vi "HXG2_PIDs_Array_Industrial.vi"(0 "Calculated Values":T3, 1 "PID Cluster":T7, 2 "Evap Target Delta (-°F) 2":cluster{"m":dbl, "b":dbl}={"m"=0.2667, "b"=7.333}, 3 "AIR-LIQ Cluster":T4 {"Liq Cluster"."Liq TEMP %" min=0.0 max=100.0 step=1.0 format="%#.1f"; "Liq Cluster"."Liq FLOW %" min=0.0 max=100.0 step=1.0 format="%#.1f"; "Liq Cluster"."TLiq °F" min=40.0 max=180.0 step=1.0 format="%#.1f"; "Liq Cluster"."Mdot lbm/hr" min=0.0 max=1000.0 step=1.0 format="%#.1f"; "Air Cluster"."Air TEMP %" min=0.0 max=100.0 step=1.0 format="%#.1f"; "Air Cluster"."Air FLOW %" min=0.0 max=100.0 step=1.0 format="%#.1f"; "Air Cluster"."Tair  °F" min=-5.0 max=100.0 step=1.0 format="%#.1f"; "Air Cluster"."CFMs" min=0.0 max=200.0 step=1.0 format="%#.1f"}, 4 "Tank Target Delta (+°F)":dbl, 5 "error in (no error)":errorcluster, 6 "Analog In":T2, 7 "PID Ctrls":T1) -> (14 "PID Ctrls Out":T1, 19 "error out":errorcluster)   [LabVIEW 2012]
uses:
  Controls/HXG2_PIDctrlsOUT.ctl
  Controls/HXG2_PIDCluster.ctl
  Controls/HXG2_PIDon-off.ctl
  PID/HXG2_Horizontal PID Control.ctl
  PID/HXG2_Horizontal Reset Control.ctl
  Controls/HXG2_AirGly-Cluster.ctl
  Controls/UI/HXG2_UI_ControlSetAir.ctl
  Controls/UI/HXG2_UI_ControlSetGly.ctl
  Controls/HXG2_Calculated.ctl
  Controls/HXG2_AnalogIn.ctl
  Modules/EnableAirGly/HXG2enable.ctl
  Controls/UI/HXG2_NumDisplayLarge.ctl
  <vilib>/addons/control/pid/pid.llb/PID Advanced (DBL Array).vi
  <vilib>/addons/control/pid/pid.llb/PID Derivative Action Buffered (DBL Array).vi
  <vilib>/addons/control/pid/pid.llb/PID Get Advanced Error (DBL Array).vi
  <vilib>/addons/control/pid/pid.llb/PID Integral Action Buffered (DBL Array).vi
  <vilib>/addons/control/pid/pid.llb/PID Resize 1D Array.vi
  <vilib>/addons/control/pid/pid.llb/PID Get Advanced Error (DBL).vi
  <vilib>/addons/control/pid/pid.llb/PID Control Input Filter (DBL).vi
  <vilib>/addons/control/pid/pid.llb/PID Gain Schedule (DBL).vi
  <vilib>/addons/control/pid/pid.llb/PID Parameter Manager (DBL Array).vi
  <vilib>/addons/control/pid/NI_PID_pid.lvlib
panel:
  out "index out Air":i32
  out "index out Liq":i32
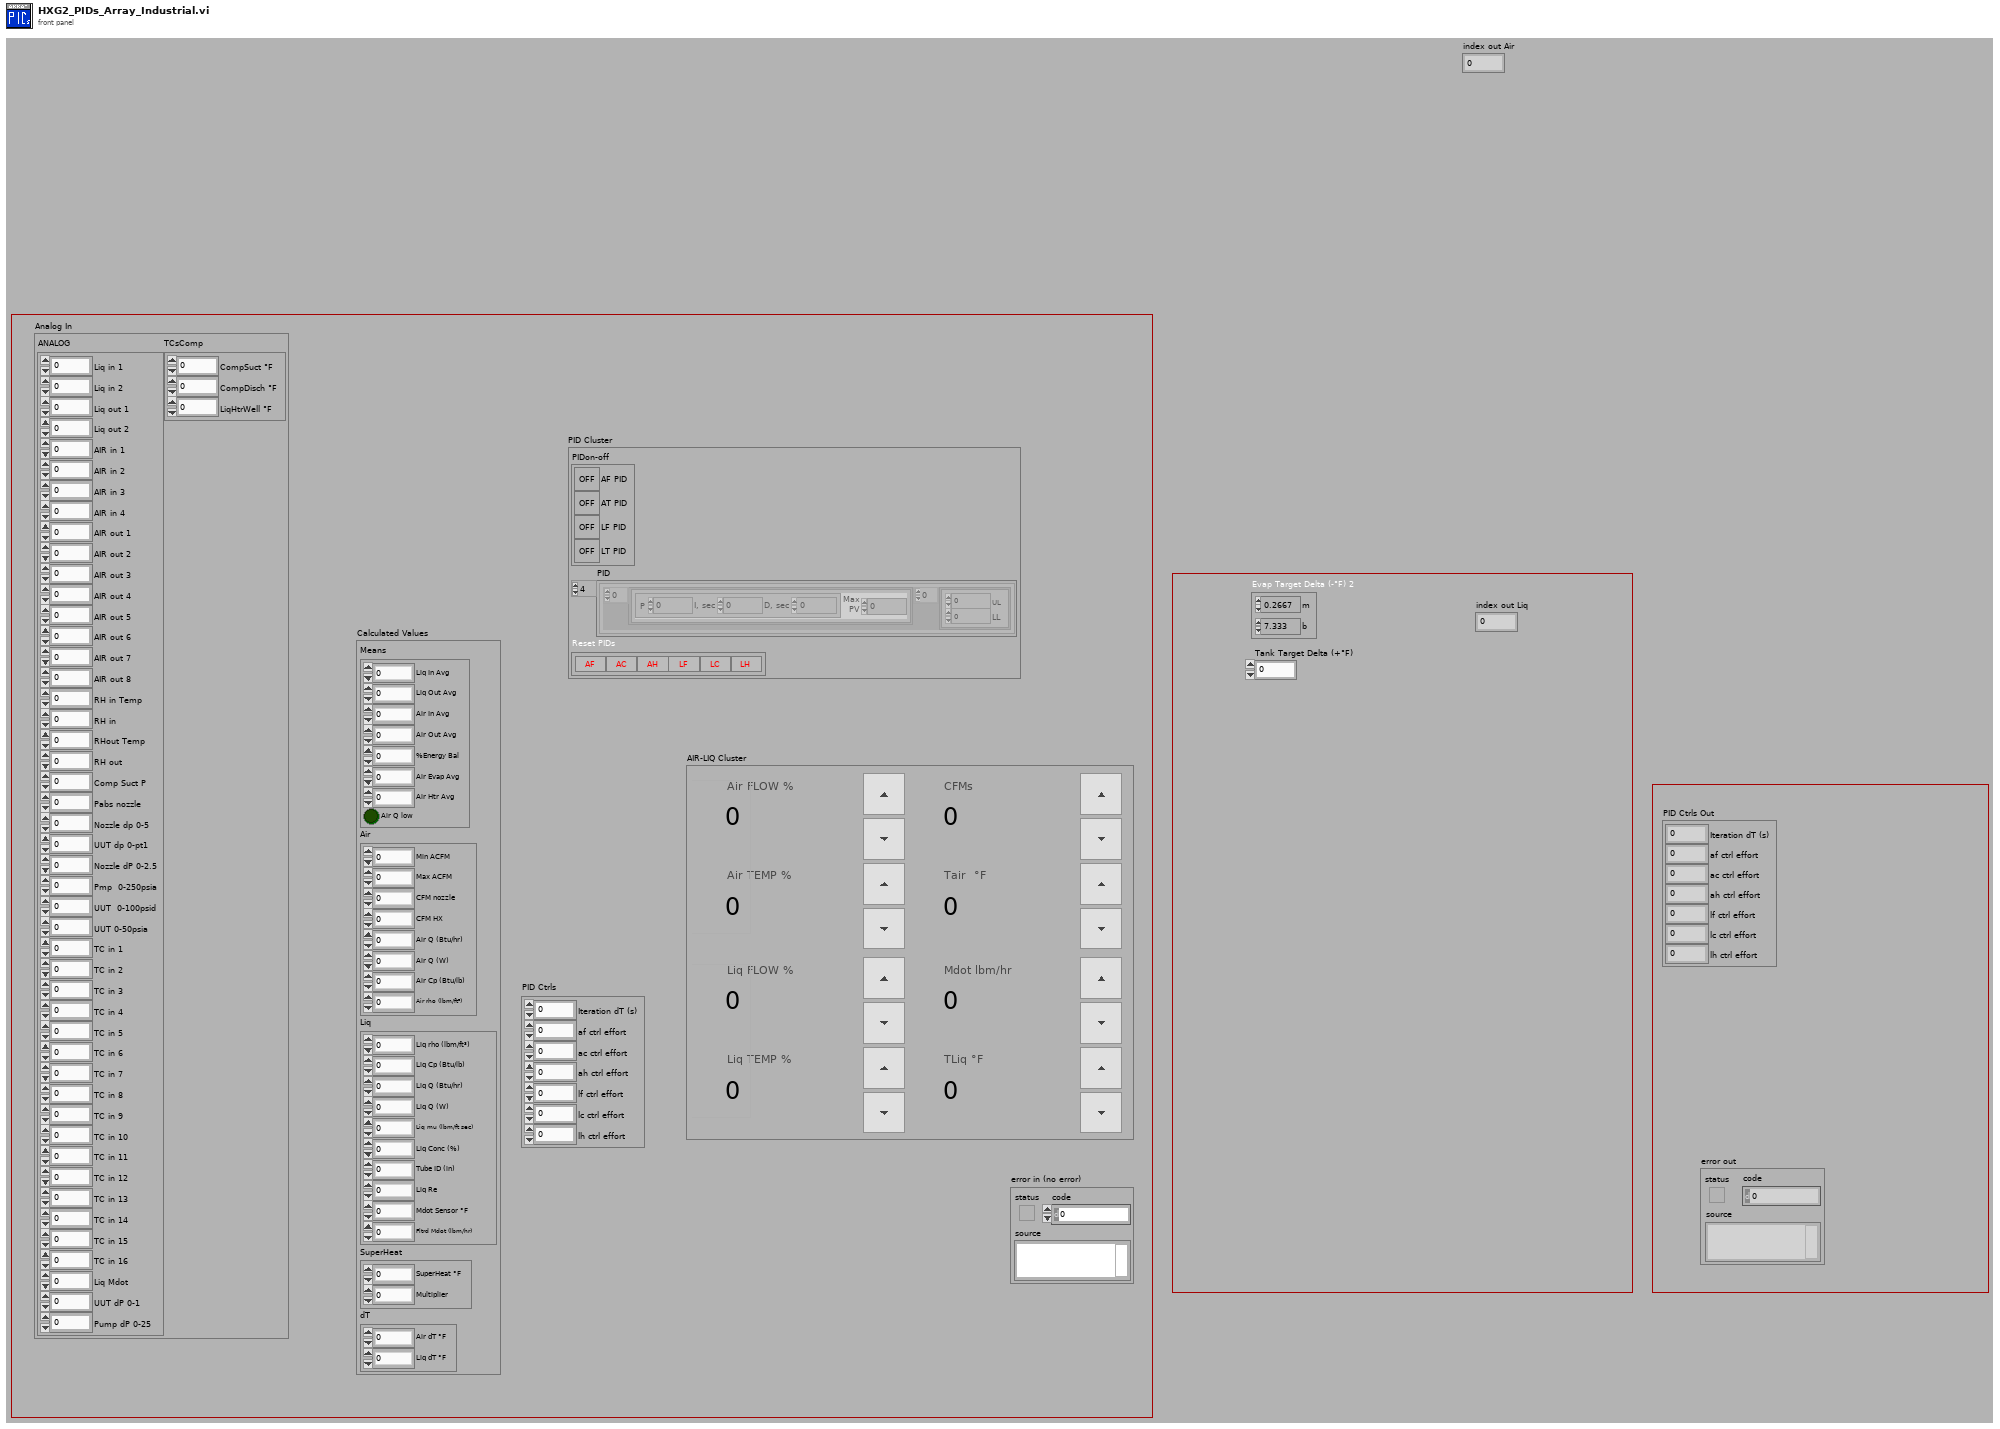
[diagram p1: front panel]
types:
  T1 = typedef "HXG2_PIDctrlsOUT.ctl" = cluster{"Iteration dT (s)":dbl, "af ctrl effort":dbl, "ac ctrl effort":dbl, "ah ctrl effort":dbl, "lf ctrl effort":dbl, "lc ctrl effort":dbl, "lh ctrl effort":dbl}
  T2 = typedef "HXG2_AnalogIn.ctl" = cluster{"ANALOG":cluster{"Liq in 1":dbl, "Liq in 2":dbl, "Liq out 1":dbl, "Liq out 2":dbl, "AIR in 1":dbl, "AIR in 2":dbl, "AIR in 3":dbl, "AIR in 4":dbl, "AIR out 1":dbl, "AIR out 2":dbl, "AIR out 3":dbl, "AIR out 4":dbl, "AIR out 5":dbl, "AIR out 6":dbl, "AIR out 7":dbl, "AIR out 8":dbl, "RH in Temp":dbl, "RH in":dbl, "RHout Temp":dbl, "RH out":dbl, "Comp Suct P":dbl, "Pabs nozzle":dbl, "Nozzle dp 0-5":dbl, "UUT dp 0-pt1":dbl, "Nozzle dP 0-2.5":dbl, "Pmp  0-250psia":dbl, "UUT  0-100psid":dbl, "UUT 0-50psia":dbl, "TC in 1":dbl, "TC in 2":dbl, "TC in 3":dbl, "TC in 4":dbl, "TC in 5":dbl, "TC in 6":dbl, "TC in 7":dbl, "TC in 8":dbl, "TC in 9":dbl, "TC in 10":dbl, "TC in 11":dbl, "TC in 12":dbl, "TC in 13":dbl, "TC in 14":dbl, "TC in 15":dbl, "TC in 16":dbl, "Liq Mdot":dbl, "UUT dP 0-1":dbl, "Pump dP 0-25":dbl}, "TCsComp":cluster{"CompSuct °F  ":dbl, "CompDisch °F":dbl, "LiqHtrWell °F":dbl}}
  T3 = typedef "HXG2_Calculated.ctl" = cluster{"Means":cluster{"Liq In Avg":dbl, "Liq Out Avg":dbl, "Air In Avg":dbl, "Air Out Avg":dbl, "%Energy Bal":dbl, "Air Evap Avg":dbl, "Air Htr Avg":dbl, "Air Q low":bool}, "Air":cluster{"Min ACFM":dbl, "Max ACFM":dbl, "CFM nozzle":dbl, "CFM HX":dbl, "Air Q (Btu/hr)":dbl, "Air Q (W)":dbl, "Air Cp (Btu/lb)":dbl, "Air rho (lbm/ft³)":dbl}, "Liq":cluster{"Liq rho (lbm/ft³)":dbl, "Liq Cp (Btu/lb)":dbl, "Liq Q (Btu/hr)":dbl, "Liq Q (W)":dbl, "Liq mu (lbm/ft sec)":dbl, "Liq Conc (%)":dbl, "Tube ID (in)":dbl, "Liq Re":dbl, "Mdot Sensor °F":dbl, "Fltrd Mdot (lbm/hr)":dbl}, "SuperHeat":cluster{"SuperHeat °F":dbl, "Multiplier":dbl}, "dT":cluster{"Air dT °F":dbl, "Liq dT °F":dbl}}
  T4 = typedef "HXG2_AirGly-Cluster.ctl" = cluster{"Air Cluster":T5, "Liq Cluster":T6}
  T5 = typedef "HXG2_UI_ControlSetAir.ctl" = cluster{"Air FLOW %":dbl, "Air TEMP % ":dbl, "CFMs":dbl, "Tair  °F":dbl}
  T6 = typedef "HXG2_UI_ControlSetGly.ctl" = cluster{"Liq FLOW %":dbl, "Liq TEMP % ":dbl, "Mdot lbm/hr":dbl, "TLiq °F":dbl}
  T7 = typedef "HXG2_PIDCluster.ctl" = cluster{"PIDon-off ":T8, "PID":T9, "Reset PIDs":T10}
  T8 = typedef "HXG2_PIDon-off.ctl" = cluster{"AF PID":bool, "AT PID":bool, "LF PID":bool, "LT PID":bool}
  T9 = typedef "HXG2_Horizontal PID Control.ctl" = cluster{"GainsArray":cluster{"Gains 2":cluster{"P":dbl, "I, sec":dbl, "D, sec":dbl}, "Max\nPV":dbl}[], "UL-LL Array":cluster{"UL":dbl, "LL  ":dbl}[]}[]
  T10 = typedef "HXG2_Horizontal Reset Control.ctl" = cluster{"AF":bool, "AC":bool, "AH":bool, "LF":bool, "LC":bool, "LH":bool}
  T11 = cluster{"setpoint high":dbl, "setpoint low":dbl}[]
  T12 = typedef "HXG2enable.ctl" = enum16{"Write Refs", "Write", "Pass"}
  T13 = typedef "HXG2_NumDisplayLarge.ctl" = dbl
  T14 = cluster{"Gains 2":cluster{"P":dbl, "I, sec":dbl, "D, sec":dbl}, "Max\nPV":dbl}[]
  T15 = cluster{"proportional gain (Kc)":dbl, "integral time (Ti, min)":dbl, "derivative time (Td, min)":dbl}
  T16 = cluster{"output[0]":dbl, "output[1]":dbl, "output[2]":dbl}
  T17 = cluster{"[0]":dbl, "[1]":dbl, "[2]":dbl, "[3]":dbl}
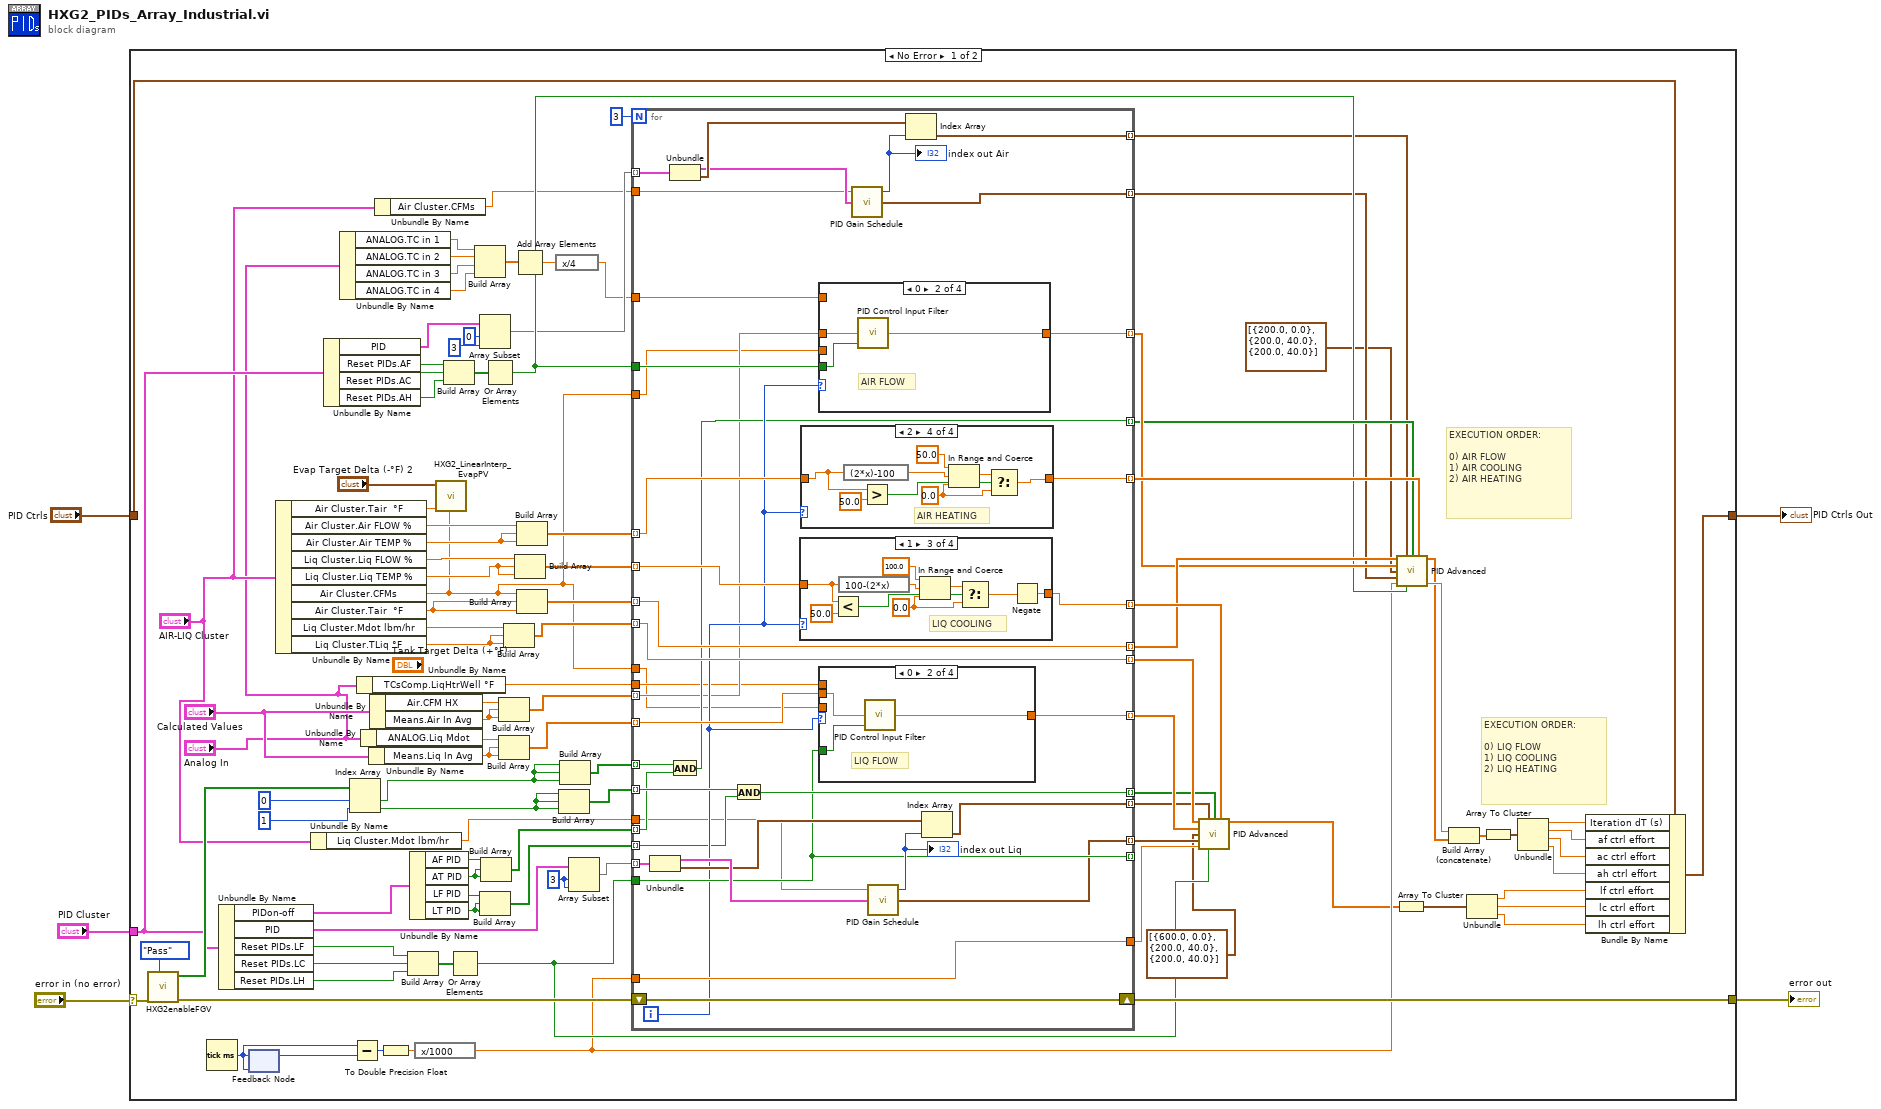
[diagram p0: block diagram]
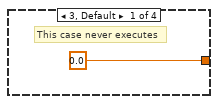
[diagram p2: hidden frame]
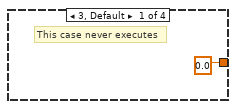
[diagram p5: hidden frame]
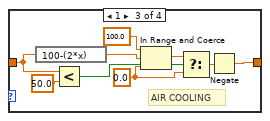
[diagram p7: hidden frame]
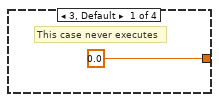
[diagram p8: hidden frame]
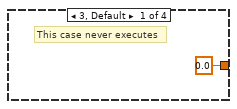
[diagram p11: hidden frame]
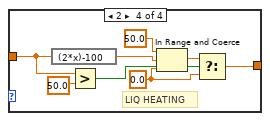
[diagram p13: hidden frame]
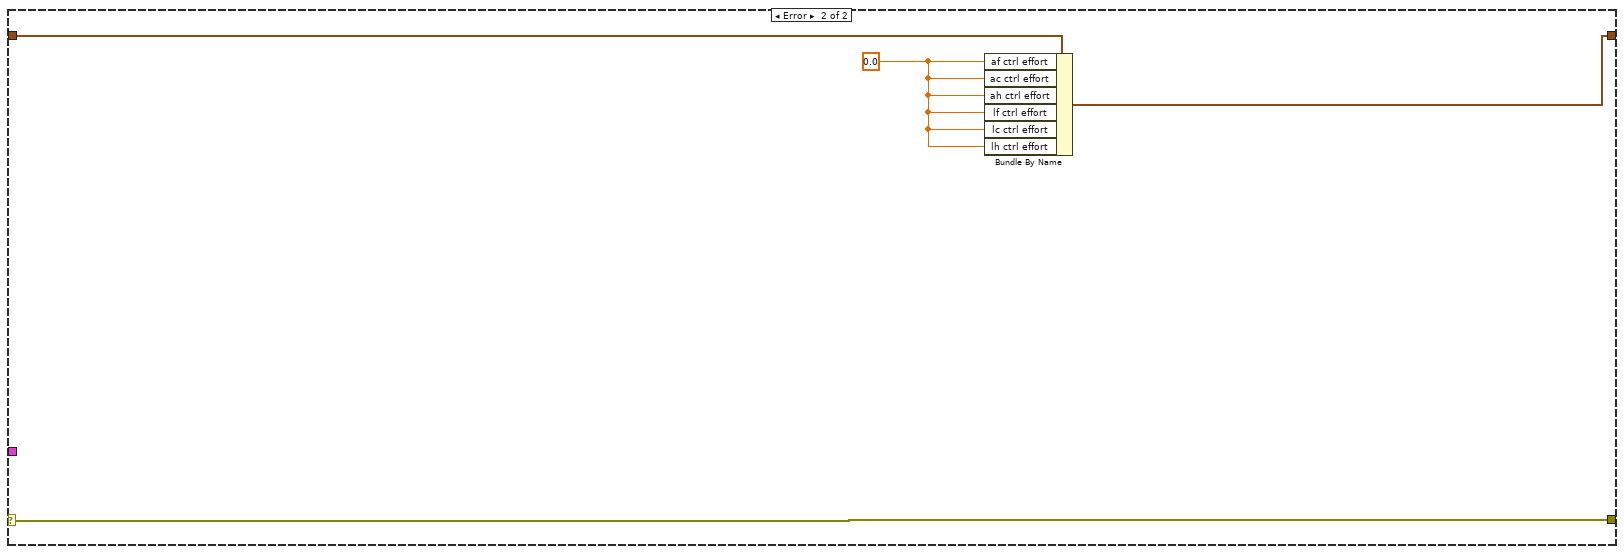
[diagram p14: hidden frame]
diagram:
  n1 = case shown="No Error" "error in (no error)" {
    selector: "error in (no error)" -> [w110 w203]
    tunnel: [w94 w203] -> w5
    tunnel: [w92 w201] -> w2
    tunnel: "PID Ctrls" -> [w93 w202]
    tunnel: "PID Cluster" -> [w58 _]
    frame No Error {
      w46 = 3 ("index")
      # "EXECUTION ORDER:\n\n0) AIR FLOW\n1) AIR COOLING\n2) AIR HEATING"
      # "EXECUTION ORDER:\n\n0) LIQ FLOW\n1) LIQ COOLING\n2) LIQ HEATING"
      n2 = call "HXG2enableFGV.vi"("ENABLE Ctrl"=HXG2enable."Pass", "error in (no error)"=w110) -> ("error out"=w95:errorcluster, "Air-Liq Out"=w97:bool[])  [unwired: 7 in, 1 out]
      n3 = Tick Count (ms)() -> (millisecond timer value=w103:u32)
      n4 = Unbundle By Name(w58) -> ("PIDon-off"=w90:T8, "PID"=w47:T9, "Reset PIDs.LF"=w53:bool, "Reset PIDs.LC"=w52:bool, "Reset PIDs.LH"=w51:bool)
      n5 = feedback #1(w103) -> (w101:u32)
      n6 = feedback-in #1(w103) -> ()
      n7 = Unbundle By Name("AIR-LIQ Cluster") -> ("Air Cluster.Tair  °F"=w9:dbl, "Air Cluster.Air FLOW %"=w81:dbl, "Air Cluster.Air TEMP %"=w80:dbl, "Liq Cluster.Liq FLOW %"=w107:dbl, "Liq Cluster.Liq TEMP %"=w106:dbl, "Air Cluster.CFMs"=w10:dbl, "Air Cluster.Tair  °F"=w8:dbl, "Liq Cluster.Mdot lbm/hr"=w24:dbl, "Liq Cluster.TLiq °F"=w7:dbl)
      n8 = Unbundle By Name("AIR-LIQ Cluster") -> ("Liq Cluster.Mdot lbm/hr"=w21:dbl)
      n9 = Unbundle By Name(w58) -> ("PID"=w43:T9, "Reset PIDs.AF"=w57:bool, "Reset PIDs.AC"=w56:bool, "Reset PIDs.AH"=w55:bool)
      n10 = Unbundle By Name("Analog In") -> ("ANALOG.TC in 1"=w20:dbl, "ANALOG.TC in 2"=w19:dbl, "ANALOG.TC in 3"=w18:dbl, "ANALOG.TC in 4"=w17:dbl)
      n11 = Index Array(array=w97, index #1=0 ("index"), index #2=1 ("index")) -> (element #1=w67:bool, element #2=w98:bool)
      n12 = Subtract(x=w103, y=w101) -> (x-y=w102:u32)
      n13 = Unbundle By Name("Analog In") -> ("TCsComp.LiqHtrWell °F"=w12:dbl)
      n14 = Unbundle By Name("Analog In") -> ("ANALOG.Liq Mdot"=w72:dbl)
      n15 = Unbundle By Name("Calculated Values") -> ("Means.Liq In Avg"=w71:dbl)
      n16 = Unbundle By Name("Calculated Values") -> ("Air.CFM HX"=w74:dbl, "Means.Air In Avg"=w73:dbl)
      n17 = Unbundle By Name("AIR-LIQ Cluster") -> ("Air Cluster.CFMs"=w23:dbl)
      n18 = To Double Precision Float(number=w102) -> (double precision float=w104:dbl)
      n19 = Build Array(w53, w52, w51) -> (w50:bool[])
      n20 = Unbundle By Name(w90) -> ("AF PID"=w63:bool, "AT PID"=w62:bool, "LF PID"=w64:bool, "LT PID"=w61:bool)
      n21 = expression code="x/1000"(w104) -> (w38:dbl)
      n22 = call "HXG2_LinearInterp_EvapPV.vi"("CFM"=w10, "Tair  °F"=w9, "Evap Target Delta (-°F) in"="Evap Target Delta (-°F) 2") -> ()  [unwired: 8 in, 1 out]
      n23 = Build Array(w57, w56, w55) -> (w54:bool[])
      n24 = Or Array Elements(Boolean array=w50) -> (logical OR=w49:bool)
      n25 = Build Array(w20, w19, w18, w17) -> (w16:dbl[])
      n26 = Array Subset(array=w43, index=0, length=3 ("index")) -> (w41:T9)
      n27 = Build Array(w64, w61, w61) -> (w60:bool[])
      n28 = Build Array(w63, w62, w62) -> (w59:bool[])
      n29 = Or Array Elements(Boolean array=w54) -> (logical OR=w48:bool)
      n30 = Build Array(w74, w73, w73) -> (w69:dbl[])
      n31 = Build Array(w72, w71, w71) -> (w70:dbl[])
      n32 = Build Array(w24, w7, w7) -> (w75:dbl[])
      n33 = Add Array Elements(numeric array=w16) -> (sum=w15:dbl)
      n34 = Build Array(w107, w106, w106) -> (w105:dbl[])
      n35 = Build Array(w81, w80, w80) -> (w79:dbl[])
      n36 = Build Array(w10, w8, w8) -> (w77:dbl[])
      n37 = expression code="x/4"(w15) -> (w14:dbl)
      n38 = Build Array(w98, w98, w98) -> (w96:bool[])
      n39 = Build Array(w67, w67, w67) -> (w66:bool[])
      n40 = Array Subset(array=w47, index=w46, length=w46) -> (w45:T9)
      n41 = for {
        N: 3 -> [_]
        tunnel: w60 -> [w129] mode=indexing
        tunnel: w70 -> [w145] mode=indexing
        tunnel: w75 -> [w141] mode=indexing
        tunnel: w105 -> [w146] mode=indexing
        tunnel: w38 -> [w137]
        tunnel: w96 -> [w149] mode=indexing
        tunnel: w45 -> [w148] mode=indexing
        shift-right: [w147] -> w94
        shift-left: w95 -> [w147]
        tunnel: w49 -> [w136]
        tunnel: [w141] -> w89 mode=indexing
        tunnel: [w140] -> w88 mode=indexing
        tunnel: [w139] -> w87 mode=indexing
        tunnel: [w138] -> w86 mode=indexing
        tunnel: [w135] -> w85 mode=indexing
        tunnel: [w112] -> w84 mode=indexing
        tunnel: [w137] -> w83
        tunnel: [w136] -> _ mode=indexing
        tunnel: w79 -> [w134] mode=indexing
        tunnel: [w133] -> w78 mode=indexing
        tunnel: w77 -> [w132] mode=indexing
        tunnel: [w132] -> w76 mode=indexing
        tunnel: w69 -> [w120] mode=indexing
        tunnel: [w131] -> w68 mode=indexing
        tunnel: w66 -> [w128] mode=indexing
        tunnel: [w127] -> w65 mode=indexing
        tunnel: w59 -> [w126] mode=indexing
        tunnel: w48 -> [w125]
        tunnel: w41 -> [w123] mode=indexing
        tunnel: [w111] -> w40 mode=indexing
        tunnel: [w119] -> w39 mode=indexing
        tunnel: w23 -> [w118]
        tunnel: w21 -> [w117]
        tunnel: w14 -> [w116]
        tunnel: w12 -> [w115]
        tunnel: w10 -> [w114]
        tunnel: w10 -> [w113]
        i -> [w130]
        n42 = Unbundle(w148) -> ("GainsArray"=w143:T14, "UL-LL Array"=w142:cluster{"UL":dbl, "LL  ":dbl}[])
        n43 = Unbundle(w123) -> ("GainsArray"=w121:T14, "UL-LL Array"=w122:cluster{"UL":dbl, "LL  ":dbl}[])
        n44 = And(x=w128, y=w126) -> (x .and. y?=w127:bool)
        n45 = And(x=w149, y=w129) -> (x .and. y?=w138:bool)
        n46 = case shown="1" w130 {
          tunnel: w146 -> [_ w182 w184 w194]
          tunnel: [0.0 ("Liq In Avg") w182 w183 w192] -> w139
          frame 3, Default {
            # "This case never executes"
          }
          frame 0 {
            # "LIQ FLOW"
          }
          frame 1 {
            w187 = T13 0.0 ("lower limit")
            # "LIQ COOLING"
            n47 = Less?(x=w184, y=T13 50.0) -> (x < y?=w186:bool)
            n48 = expression code="100-(2*x)"(w184) -> (w189:dbl)
            n49 = In Range and Coerce(upper limit=T13 100.0, x=w189, lower limit=w187) -> (coerced(x)=w190:T13)  [unwired: 1 out]
            n50 = Select(t=w190, s=w186, f=w187) -> (s? t:f=w191:T13)
            n51 = Negate(x=w191) -> (-x=w183:T13)
          }
          frame 2 {
            w199 = T13 0.0 ("lower limit")
            # "LIQ HEATING"
            n52 = expression code="(2*x)-100"(w194) -> (w197:dbl)
            n53 = Greater?(x=w194, y=T13 50.0) -> (0:w195:bool)
            n54 = In Range and Coerce(upper limit=T13 50.0, x=w197, lower limit=w199) -> (coerced(x)=w198:T13)  [unwired: 1 out]
            n55 = Select(t=w198, s=w195, f=w199) -> (s? t:f=w192:T13)
          }
        }
        n56 = case shown="2" w130 {
          tunnel: w134 -> [_ w157 w160 w169]
          tunnel: [0.0 ("Liq In Avg") w157 w158 w167] -> w133
          frame 3, Default {
            # "This case never executes"
          }
          frame 0 {
            # "AIR FLOW"
          }
          frame 1 {
            w162 = T13 0.0 ("lower limit")
            # "AIR COOLING"
            n57 = expression code="100-(2*x)"(w160) -> (w163:dbl)
            n58 = Less?(x=w160, y=T13 50.0) -> (x < y?=w161:bool)
            n59 = In Range and Coerce(upper limit=T13 100.0, x=w163, lower limit=w162) -> (coerced(x)=w164:T13)  [unwired: 1 out]
            n60 = Select(t=w164, s=w161, f=w162) -> (s? t:f=w166:T13)
            n61 = Negate(x=w166) -> (-x=w158:T13)
          }
          frame 2 {
            w174 = T13 0.0 ("lower limit")
            # "AIR HEATING"
            n62 = expression code="(2*x)-100"(w169) -> (w172:dbl)
            n63 = Greater?(x=w169, y=T13 50.0) -> (0:w170:bool)
            n64 = In Range and Coerce(upper limit=T13 50.0, x=w172, lower limit=w174) -> (coerced(x)=w173:T13)  [unwired: 1 out]
            n65 = Select(t=w173, s=w170, f=w174) -> (s? t:f=w167:T13)
          }
        }
        n66 = case shown="0" w130 {
          tunnel: w120 -> [_ w153 w154 w155]
          tunnel: [0.0 ("Liq In Avg") w152 w154 w155] -> w131
          tunnel: w125 -> [_ w151 _ _]
          tunnel: w116 -> [_ _ _ _]
          tunnel: w114 -> [_ _ _ _]
          frame 3, Default {
            # "This case never executes"
          }
          frame 0 {
            # "AIR FLOW"
            n67 = call-poly <vilib>:"PID Control Input Filter.vi"("reinitialize? (F)"=w151, "input"=w153) -> ("output"=w152:dbl)  [unwired: 3 in]
          }
          frame 1 {
            # "Less than 100cfm\nTair PV is TCs else RTDs"
            # "AIR COOLING"
          }
          frame 2 {
            # "AIR HEATING"
          }
        }
        n68 = case shown="0" w130 {
          tunnel: w145 -> [_ w178 w179 w180]
          tunnel: [0.0 ("Liq In Avg") w176 w179 w180] -> w140
          tunnel: w136 -> [_ w177 _ _]
          tunnel: w115 -> [_ _ _ _]
          tunnel: w113 -> [_ _ _ _]
          frame 3, Default {
            # "This case never executes"
          }
          frame 0 {
            # "LIQ FLOW"
            n69 = call-poly <vilib>:"PID Control Input Filter.vi"("reinitialize? (F)"=w177, "input"=w178) -> ("output"=w176:dbl)  [unwired: 3 in]
          }
          frame 1 {
            # "LIQ COOLING"
          }
          frame 2 {
            # "LIQ HEATING"
          }
        }
        n70 = call-poly <vilib>:"PID Gain Schedule.vi"("PID gain schedule"=w121, "gain scheduling value"=w118) -> ("PID gains out"=w111:T15, "index out"=w124:i32)  [unwired: 2 in]
        "index out Air" <- w124
        n71 = call-poly <vilib>:"PID Gain Schedule.vi"("PID gain schedule"=w143, "gain scheduling value"=w117) -> ("PID gains out"=w112:T15, "index out"=w144:i32)  [unwired: 2 in]
        "index out Liq" <- w144
        n72 = Index Array(array=w122, index=w124) -> (element=w119:cluster{"UL":dbl, "LL  ":dbl})
        n73 = Index Array(array=w142, index=w144) -> (element=w135:cluster{"UL":dbl, "LL  ":dbl})
      }
      n74 = call-poly <vilib>:"PID Advanced.vi"("setpoint"=w89, "output range"=w85, "auto? (T)"=w86, "manual control"=w87, "process variable"=w88, "setpoint range"=T11 [{"setpoint high"=600.0, "setpoint low"=0.0}, {"setpoint high"=200.0, "setpoint low"=40.0}, {"setpoint high"=200.0, "setpoint low"=40.0}], "PID gains"=w84, "dt (s)"=w83, "reinitialize? (F)"=w49) -> ("output"=w37:dbl[])  [unwired: 5 in, 1 out]
      n75 = Array To Cluster(array=w37) -> (cluster=w91:T16)
      n76 = call-poly <vilib>:"PID Advanced.vi"("setpoint"=w76, "output range"=w39, "auto? (T)"=w65, "manual control"=w78, "process variable"=w68, "setpoint range"=T11 [{"setpoint high"=200.0, "setpoint low"=0.0}, {"setpoint high"=200.0, "setpoint low"=40.0}, {"setpoint high"=200.0, "setpoint low"=40.0}], "PID gains"=w40, "dt (s)"=w38, "reinitialize? (F)"=w48) -> ("output"=w32:dbl[], "dt out (s)"=w33:dbl)  [unwired: 5 in]
      n77 = Build Array (concatenate)(w33, w32) -> (w31:dbl[])
      n78 = Unbundle(w91) -> ("output[0]"=w36:dbl, "output[1]"=w35:dbl, "output[2]"=w34:dbl)
      n79 = Array To Cluster(array=w31) -> (cluster=w30:T17)
      n80 = Unbundle(w30) -> ("[0]"=w29:dbl, "[1]"=w28:dbl, "[2]"=w6:dbl, "[3]"=w27:dbl)
      n81 = Bundle By Name(cluster=w93, "Iteration dT (s)"=w29, "af ctrl effort"=w28, "ac ctrl effort"=w6, "ah ctrl effort"=w27, "lf ctrl effort"=w36, "lc ctrl effort"=w35, "lh ctrl effort"=w34) -> (w92:T1)
    }
    frame Error {
      w200 = 0.0 ("af ctrl effort")
      n82 = Bundle By Name(cluster=w202, "af ctrl effort"=w200, "ac ctrl effort"=w200, "ah ctrl effort"=w200, "lf ctrl effort"=w200, "lc ctrl effort"=w200, "lh ctrl effort"=w200) -> (w201:T1)
    }
  }
  "error out" <- w5
  "PID Ctrls Out" <- w2
